vi "Temp Control Message Log.vi"(7 "init?":bool, 8 "error in (no error)":errorcluster, 10 "Log Ref":refnum<vi>, 11 "String in":string) -> (0 "error out":errorcluster, 3 "Log":string)   [LabVIEW 2024]
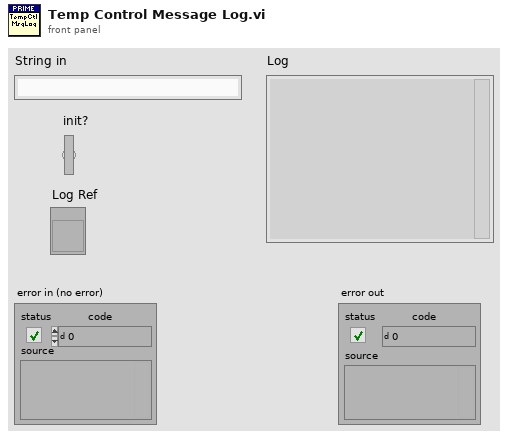
[diagram p1: front panel]
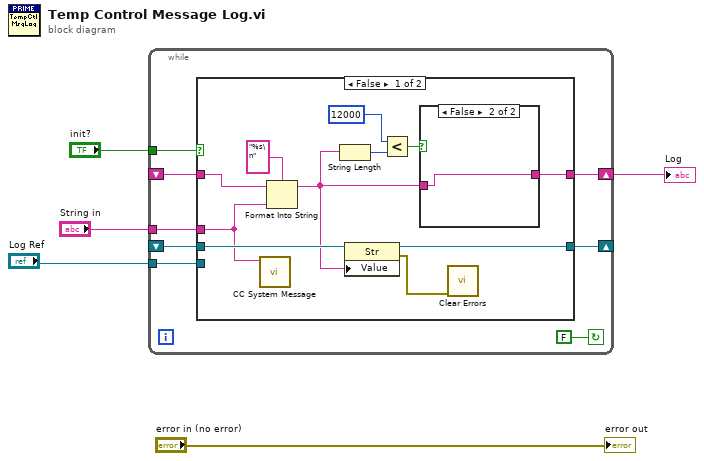
[diagram p0: block diagram]
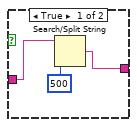
[diagram p2: hidden frame]
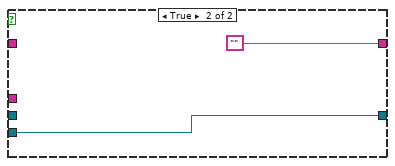
[diagram p3: hidden frame]
diagram:
  n1 = while {
    tunnel: "init?" -> [w12]
    shift-right: [w7] -> _
    shift-left: _ -> [w6]
    shift-right: [w11] -> w1
    shift-left: _ -> [w9]
    tunnel: "Log Ref" -> [w10]
    tunnel: "String in" -> [w8]
    stop <- FALSE continue-if-true
    n2 = case shown="False" w12 {
      tunnel: [w14 ""] -> w11
      tunnel: w10 -> [_ w29]
      tunnel: w9 -> [w23 _]
      tunnel: w8 -> [w19 _]
      tunnel: [w21 w29] -> w7
      tunnel: w6 -> [w22 _]
      frame False {
        n3 = call "CC System Message.vi"("Message"=w19) -> ()  [unwired: 10 in, 1 out]
        n4 = Format Into String(format string="%s\n", initial string=w23, w19) -> (resulting string=w17:string)  [unwired: 1 in, 1 out]
        n5 = String Length(string=w17) -> (length=w16:i32)
        n6 = property class="Str"(reference=w22, "Value"=w17) -> (reference out=w21:refnum<vi>, error out=w20:errorcluster)  [unwired: 1 in]
        n7 = Less?(x=12000 ("y"), y=w16) -> (x < y?=w18:bool)
        n8 = case shown="False" w18 {
          tunnel: w17 -> [w27 w28]
          tunnel: [w25 w28] -> w14
          frame True {
            n9 = Search/Split String(string=w27, offset (0)=500) -> (match + rest of string=w25:string)  [unwired: 1 in, 2 out]
          }
          frame False {
          }
        }
        n10 = call <vilib>:"Clear Errors.vi"("error in (no error)"=w20) -> ()  [unwired: 5 in, 2 out]
      }
      frame True {
      }
    }
  }
  "Log" <- w1
  "error out" <- "error in (no error)"
